vi "Decode SSL Wrapper Package.vi"(5 "Version":string(combo)="Auto", 8 "error in (no error)":errorcluster, 9 "FIRASim?":bool=TRUE, 10 "Ignore left/rigth?":bool[](array[boolean]), 11 "unsigned byte array":u8[](array[numeric])) -> (0 "error out":errorcluster, 1 "SSL_BallModelStraightTwoPhase":T1, 2 "Field Size":T2, 3 "Detection Frame":T4 {"robots_blue"."height" format="%+4.3f"; "robots_blue"."pixel_y" format="%+4.3f"; "robots_blue"."pixel_x" format="%+4.3f"; "robots_blue"."orientation" format="%+4.3f"; "robots_blue"."y" format="%+4.3f"; "robots_blue"."confidence" format="%4.3f"; "robots_blue"."x" format="%+4.3f"; "robots_yellow"."height" format="%+4.3f"; "robots_yellow"."pixel_y" format="%+4.3f"; "robots_yellow"."pixel_x" format="%+4.3f"; "robots_yellow"."orientation" format="%+4.3f"; "robots_yellow"."y" format="%+4.3f"; "robots_yellow"."confidence" format="%4.3f"; "robots_yellow"."x" format="%+4.3f"}, 4 "Empty Field Size?":bool, 6 "Empty Information?":bool)   [LabVIEW 2023]
uses:
  Controls/SSL Detection Frame.ctl
  Controls/SSL Detection Robot.ctl
  <vilib>/Analysis/Matrix/Datatypes/RealMatrix.ctl
  Controls/SSL Detection Ball.ctl
  Controls/SSL Geometry Camera Calibration.ctl
  Varint Decoder uint32.vi
  <vilib>/Analysis/Matrix/NI_Matrix.lvlib
  Controls/SSL_BallModelStraightTwoPhase.ctl
  Vision.lvclass
panel:
  out "Geometry Camera Calibration":T3
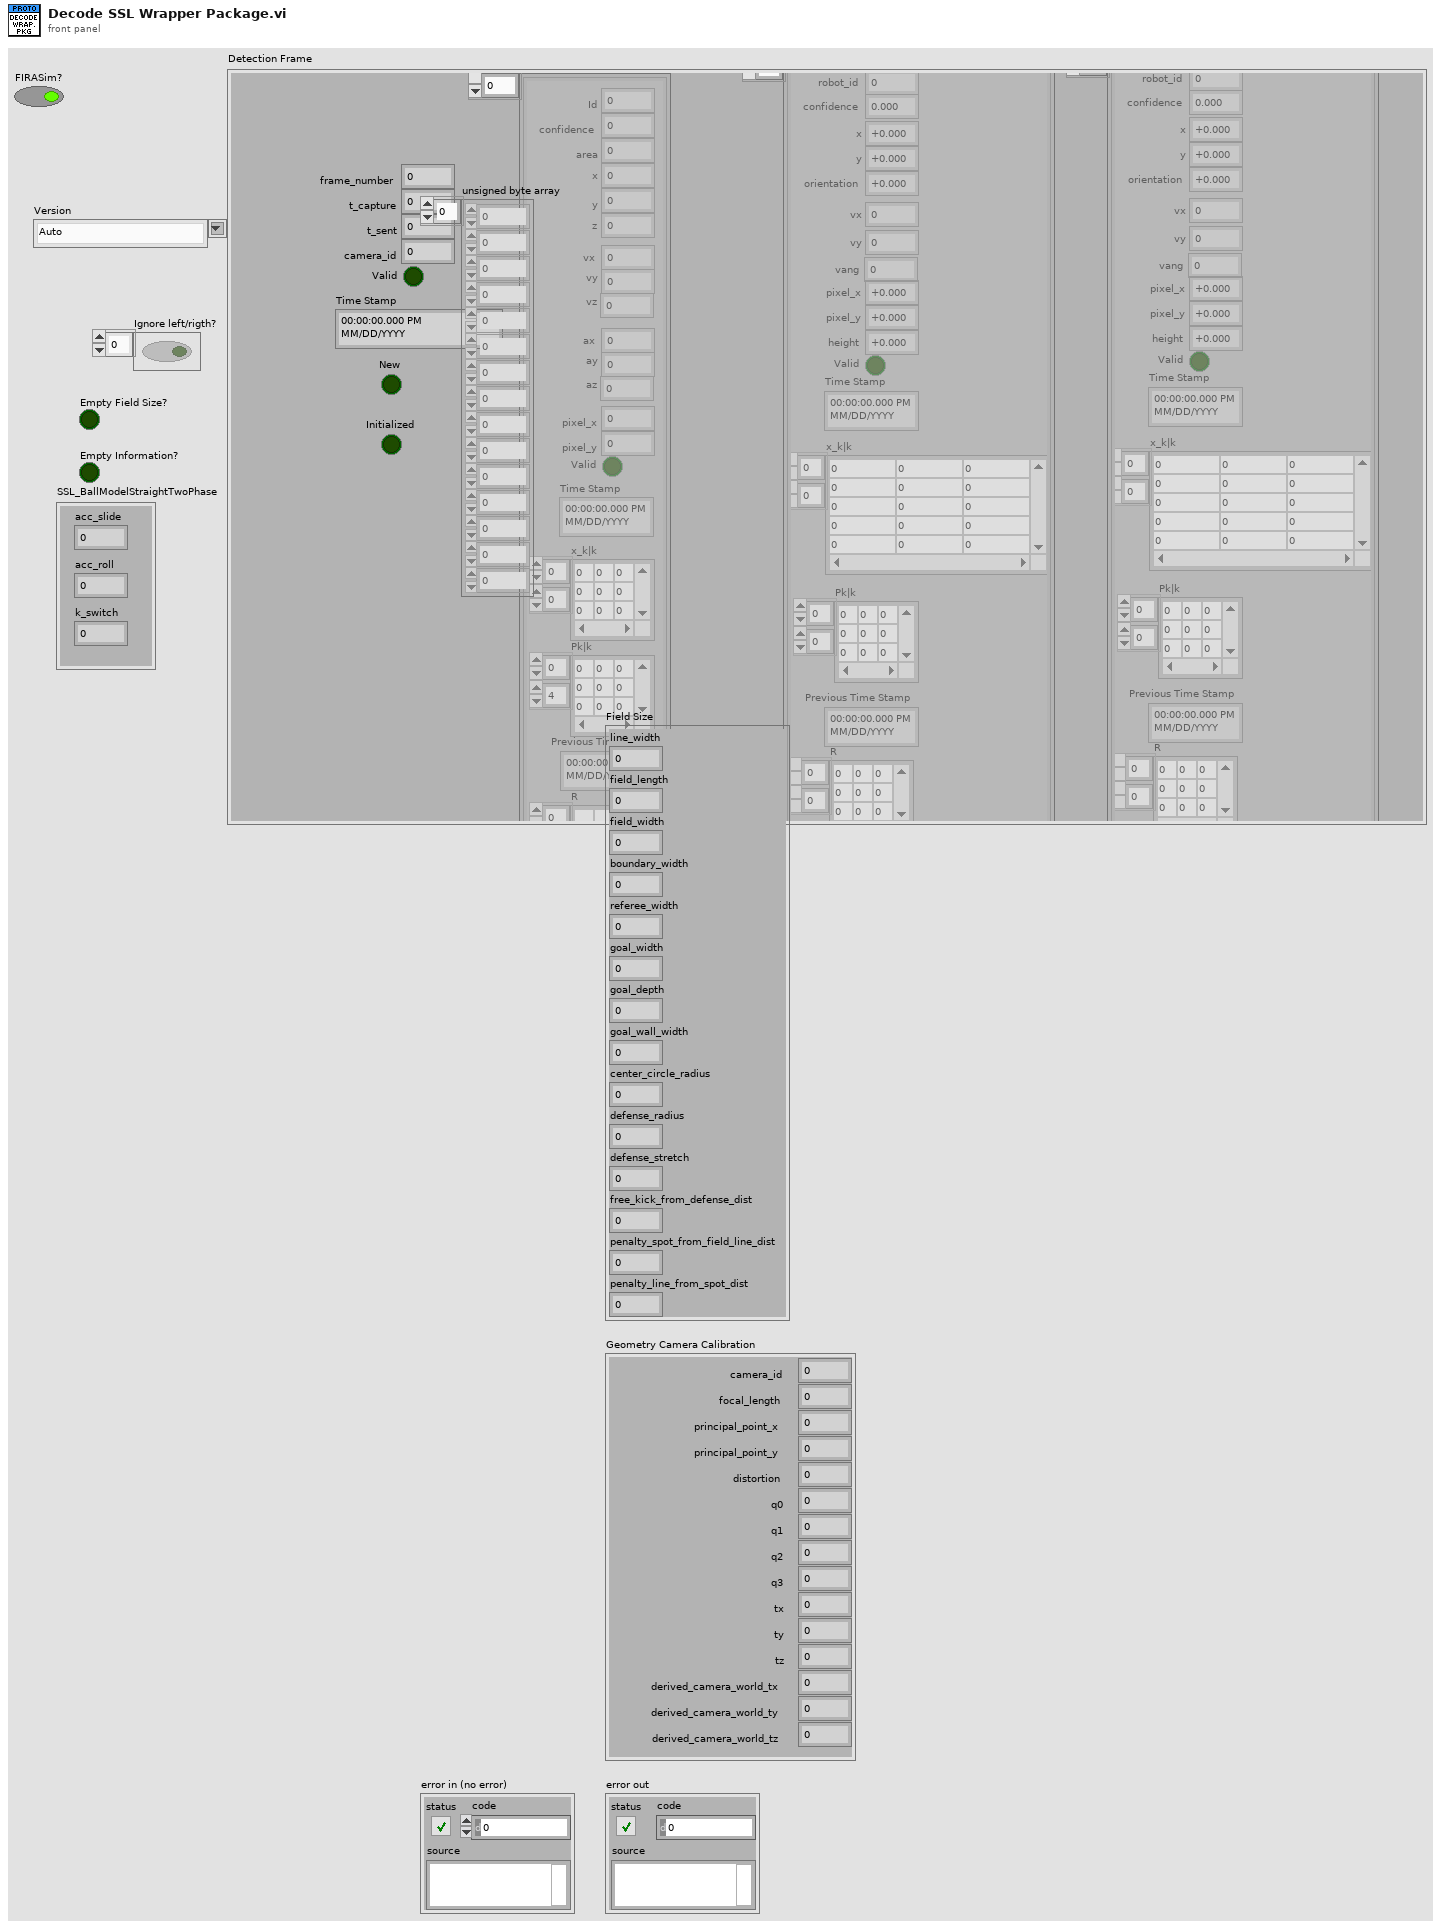
[diagram p1: front panel]
types:
  T1 = typedef "Vision.lvclass/SSL_BallModelStraightTwoPhase.ctl" = cluster{"acc_slide":dbl, "acc_roll":dbl, "k_switch":dbl}
  T2 = cluster{"line_width":u32, "field_length":u32, "field_width":u32, "boundary_width":u32, "referee_width":u32, "goal_width":u32, "goal_depth":u32, "goal_wall_width":u32, "center_circle_radius":u32, "defense_radius":u32, "defense_stretch":u32, "free_kick_from_defense_dist":u32, "penalty_spot_from_field_line_dist":u32, "penalty_line_from_spot_dist":u32}
  T3 = typedef "SSL Geometry Camera Calibration.ctl" = cluster{"camera_id":u32, "focal_length":sgl, "principal_point_x":sgl, "principal_point_y":sgl, "distortion":sgl, "q0":sgl, "q1":sgl, "q2":sgl, "q3":sgl, "tx":sgl, "ty":sgl, "tz":sgl, "derived_camera_world_tx":sgl, "derived_camera_world_ty":sgl, "derived_camera_world_tz":sgl}
  T4 = typedef "SSL Detection Frame.ctl" = cluster{"frame_number":u32, "t_capture":dbl, "t_sent":dbl, "camera_id":u32, "robots_yellow":T5[], "robots_blue":T5[], "balls":T7[], "Valid":bool, "Time Stamp":timestamp, "New":bool, "Initialized":bool}
  T5 = typedef "SSL Detection Robot.ctl" = cluster{"x":sgl, "robot_id":u32, "confidence":sgl, "y":sgl, "orientation":sgl, "pixel_x":sgl, "pixel_y":sgl, "height":sgl, "Valid":bool, "Time Stamp":timestamp, "x_k|k":T6, "Pk|k":T6, "Previous Time Stamp":timestamp, "R":T6, "vx":dbl, "vy":dbl, "vang":dbl}
  T6 = typedef "NI_Matrix.lvlib/RealMatrix.ctl" = dbl[][]
  T7 = typedef "SSL Detection Ball.ctl" = cluster{"x":sgl, "area":u32, "confidence":sgl, "y":sgl, "z":sgl, "pixel_x":sgl, "pixel_y":sgl, "Valid":bool, "Time Stamp":timestamp, "x_k|k":T6, "Pk|k":T6, "Id":u32, "Previous Time Stamp":timestamp, "R":T6, " vx":sgl, "vy":dbl, "vz":dbl, " ax":sgl, "ay":dbl, "az":dbl}
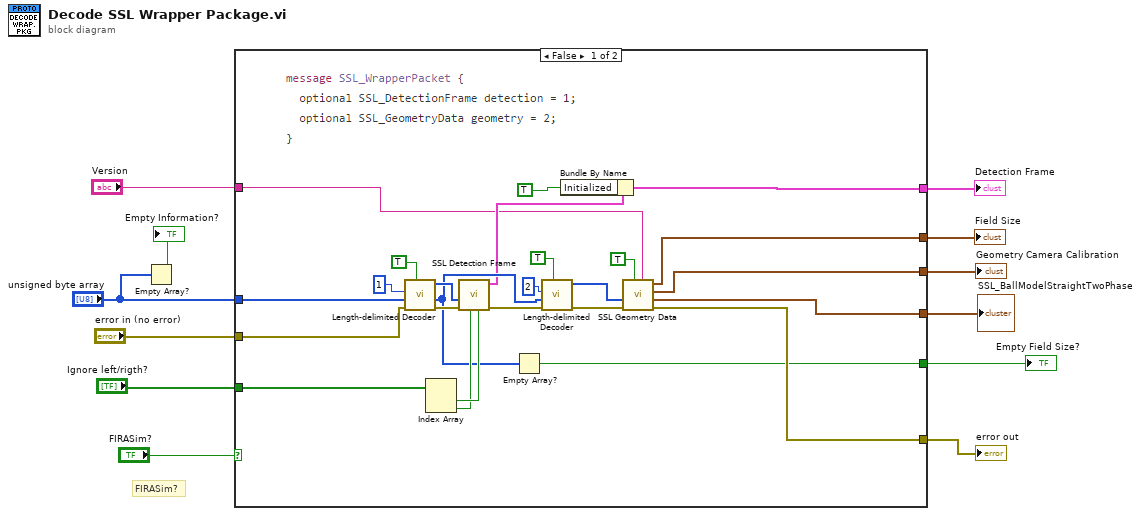
[diagram p0: block diagram]
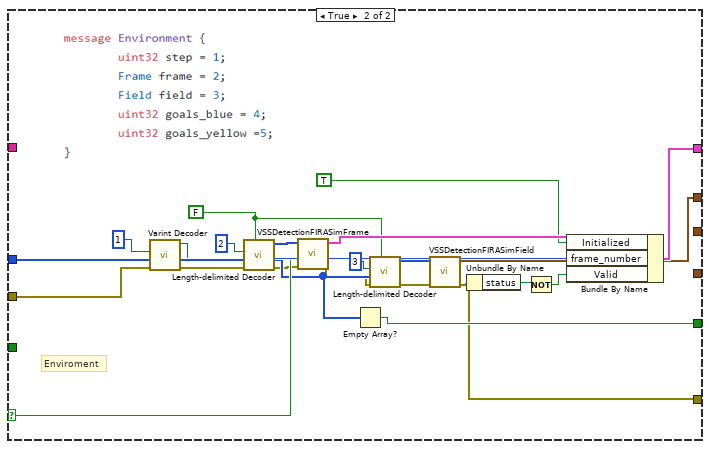
[diagram p2: hidden frame]
diagram:
  # "FIRASim?"
  n1 = Empty Array?(array="unsigned byte array") -> (empty?=→"Empty Information?":bool)
  n2 = case shown="False" "FIRASim?" {
    selector: "FIRASim?" -> [_ w53]
    tunnel: [w37 w42] -> w12
    tunnel: "Ignore left/rigth?" -> [w26 _]
    tunnel: [w23 w50] -> w5
    tunnel: [w22 _] -> w4
    tunnel: [w20 w48] -> w10
    tunnel: [w18 w54] -> w8
    tunnel: "unsigned byte array" -> [w16 w55]
    tunnel: "error in (no error)" -> [w15 w45]
    tunnel: "Version" -> [w14 _]
    tunnel: [w13 _] -> w1
    frame False {
      n3 = call "Length-delimited Decoder.vi"("Optional"=TRUE, "error in (no error)"=w15, "Array"=w16, "Key"=1) -> ("error out"=w29:errorcluster, "array w/ subset deleted"=w21:u8[], "Length-delimited"=w32:u8[])  [unwired: 4 in, 1 out]
      n4 = Index Array(array=w26) -> (element #1=w25:bool, element #2=w24:bool)  [unwired: 2 in]
      n5 = call "SSL Detection Frame.vi"("ignora esquerda?"=w25, "ignora direita?"=w24, "error in"=w29, "Array"=w32) -> ("error out"=w30:errorcluster, "Detection Frame"=w19:T4)  [unwired: 6 in]
      n6 = Empty Array?(array=w21) -> (empty?=w20:bool)
      n7 = call "Length-delimited Decoder.vi"("Optional"=TRUE, "error in (no error)"=w30, "Array"=w21, "Key"=2) -> ("error out"=w31:errorcluster, "Length-delimited"=w35:u8[])  [unwired: 4 in, 2 out]
      n8 = Bundle By Name(cluster=w19, "Initialized"=TRUE) -> (w18:T4)
      n9 = call "SSL Geometry Data.vi"("Version"=w14, "Optional"=TRUE, "error in"=w31, "Array"=w35) -> ("error out"=w37:errorcluster, "SSL_BallModelStraightTwoPhase"=w13:T1, "Geometry Camera Calibration"=w22:T3, "Field Size"=w23:T2)  [unwired: 4 in]
    }
    frame True {
      w38 = FALSE ("Optional")
      # "Enviroment"
      n10 = call-poly "Varint Decoder.vi"("error in (no error)"=w45, "Array"=w55, "Key"=1) -> ("error out"=w47:errorcluster, "array w/ subset deleted"=w60:u8[], "Varint"=w56:u32)  [unwired: 5 in, 1 out]
      n11 = call "Length-delimited Decoder.vi"("Optional"=w38, "error in (no error)"=w47, "Array"=w60, "Key"=2) -> ("error out"=w46:errorcluster, "array w/ subset deleted"=w49:u8[], "Length-delimited"=w58:u8[])  [unwired: 4 in, 1 out]
      n12 = call "VSSDetectionFIRASimFrame.vi"("error in (no error)"=w46, "FIRASim?"=w53, "Frame"=w58) -> ("error out"=w44:errorcluster, "Detection Frame out"=w57:T4)  [unwired: 7 in]
      n13 = Empty Array?(array=w49) -> (empty?=w48:bool)
      n14 = call "Length-delimited Decoder.vi"("Optional"=w38, "error in (no error)"=w44, "Array"=w49, "Key"=3) -> ("error out"=w43:errorcluster, "Length-delimited"=w51:u8[])  [unwired: 4 in, 2 out]
      n15 = call "VSSDetectionFIRASimField.vi"("error in (no error)"=w43, "Field"=w51) -> ("error out"=w42:errorcluster, "Field out"=w50:T2)  [unwired: 7 in, 1 out]
      n16 = Unbundle By Name(w42) -> ("status"=w41:bool)
      n17 = Not(x=w41) -> (.not. x?=w40:bool)
      n18 = Bundle By Name(cluster=w57, "Initialized"=TRUE, "frame_number"=w56, "Valid"=w40) -> (w54:T4)
    }
  }
  "Detection Frame" <- w8
  "error out" <- w12
  "Geometry Camera Calibration" <- w4
  "Field Size" <- w5
  "Empty Field Size?" <- w10
  "SSL_BallModelStraightTwoPhase" <- w1
